vi "Obtain Request Events.vi"(8 "error in":errorcluster, 10 "Create New? (F)":bool) -> (0 "error out":errorcluster, 2 "Full User Interface Request Events":T1)   [LabVIEW 2019, in "Full User Interface.lvlib"]
doc: "This VI Obtains/Creates the Requests events that will be used for other modules to communicate with the module that owns this VI. These Requests events will be accessed only via Public API methods for this module.\n\n<b>NOTE</b>: The contents of this VI are automatically generated and modified by the <b>Tools > DQMH Consortium > DQMH</b> utilities. Consider using those utilities instead of making your own modifications to this VI.\n_____\nBased on DQMH Project Template 7.0.1.1316."
uses:
  Full User Interface.lvlib
  Request Events--cluster.ctl
  Stop Argument--cluster.ctl
  Show Panel Argument--cluster.ctl
  Hide Panel Argument--cluster.ctl
  Get Module Execution Status Argument--cluster.ctl
  Show Diagram Argument--cluster.ctl
  Launcher Test Unit Argument--cluster.ctl
  Exit Test Unit Argument--cluster.ctl
  Load Seq Argument--cluster.ctl
  Send UUT Result Argument--cluster.ctl
  Test Unit/UUT Result.ctl
  <vilib>/Test Bench Framework/Test Executive.lvlibp/TestEngine/TestEngine/TestEngine/Typedefs/Report General.ctl
  Send User Message Argument--cluster.ctl
  Change Model Argument--cluster.ctl
  <vilib>/Test Bench Framework/Test Executive.lvlibp/TestEngine/TestEngine/TestEngine/Test Engine.lvclass
  Test Unit/Test Unit.lvlib
panel:
  # "NOTE: The contents of this VI are automatically generated and modified by the Tools > DQMH Consortium > DQMH utilities. Consider using those utilities instead of making your own modifications to this VI."
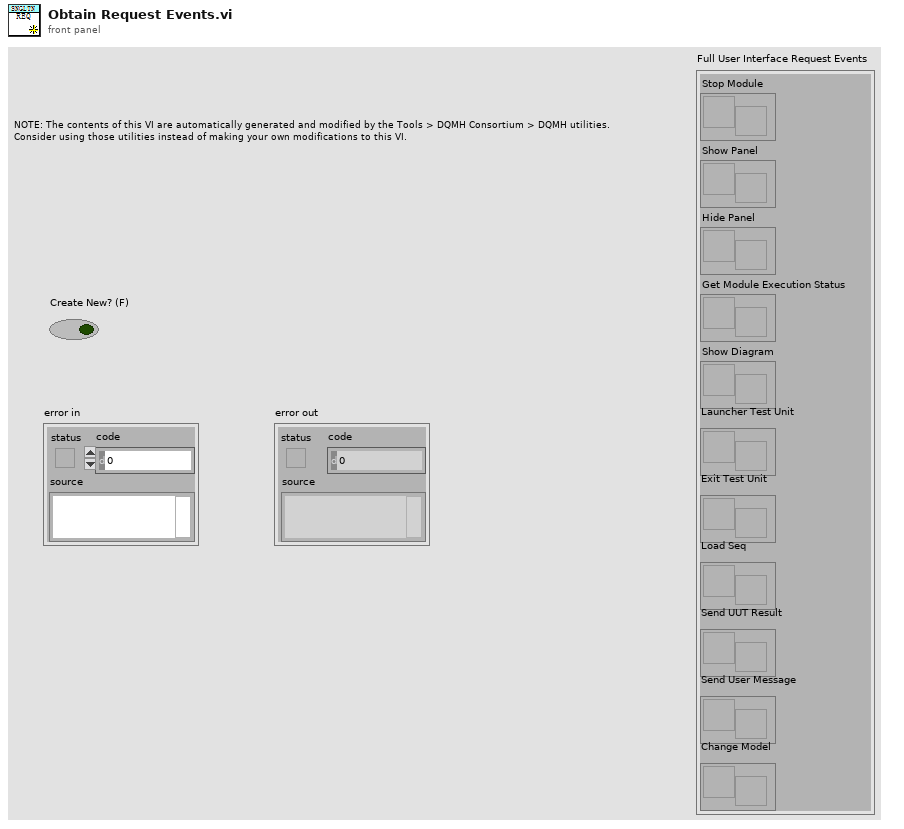
[diagram p1: front panel]
types:
  T1 = typedef "Full User Interface.lvlib/Request Events--cluster.ctl" = cluster{"Stop Module":refnum<user-event>, "Show Panel":refnum<user-event>, "Hide Panel":refnum<user-event>, "Get Module Execution Status":refnum<user-event>, "Show Diagram":refnum<user-event>, "Launcher Test Unit":refnum<user-event>, "Exit Test Unit":refnum<user-event>, "Load Seq":refnum<user-event>, "Send UUT Result":refnum<user-event>, "Send User Message":refnum<user-event>, "Change Model":refnum<user-event>}
  T2 = typedef "Full User Interface.lvlib/Change Model Argument--cluster.ctl" = cluster{"Model":string}
  T3 = typedef "Full User Interface.lvlib/Send User Message Argument--cluster.ctl" = cluster{"Station ID":i32, "Socket":i32, "UserMessage":string, "MessageData":variant}
  T4 = typedef "Full User Interface.lvlib/Send UUT Result Argument--cluster.ctl" = cluster{"UUT Result":T5, "Station":i32}
  T5 = typedef "Test Unit.lvlib/UUT Result.ctl" = cluster{"Station":i32, "Socket":i32, "DetailTestResult":string[][], "Report Path":path, "General":T6}
  T6 = typedef "Test Executive.lvlibp/Test Engine.lvlib/Test Engine.lvclass/Report General.ctl" = cluster{"Sequence Path":path, "Serial Number":string, "Test Date Time":timestamp, "UUT Status":string, "Faulty Item":string, "Seconds Executing":dbl}
  T7 = typedef "Full User Interface.lvlib/Load Seq Argument--cluster.ctl" = cluster{"Key":string}
  T8 = typedef "Full User Interface.lvlib/Exit Test Unit Argument--cluster.ctl" = cluster{"Checkbox":bool}
  T9 = typedef "Full User Interface.lvlib/Launcher Test Unit Argument--cluster.ctl" = cluster{"Checkbox":bool}
  T10 = typedef "Full User Interface.lvlib/Hide Panel Argument--cluster.ctl" = cluster{"Hide Panel?":bool}
  T11 = typedef "Full User Interface.lvlib/Show Panel Argument--cluster.ctl" = cluster{"Show Panel?":bool}
  T12 = typedef "Full User Interface.lvlib/Show Diagram Argument--cluster.ctl" = cluster{"Debug?":bool}
  T13 = typedef "Full User Interface.lvlib/Get Module Execution Status Argument--cluster.ctl" = cluster{"Running?":bool}
  T14 = typedef "Full User Interface.lvlib/Stop Argument--cluster.ctl" = cluster{"Origin":string, "Exit via Stop Module Req?":bool, "Wait for Module to stop?":bool}
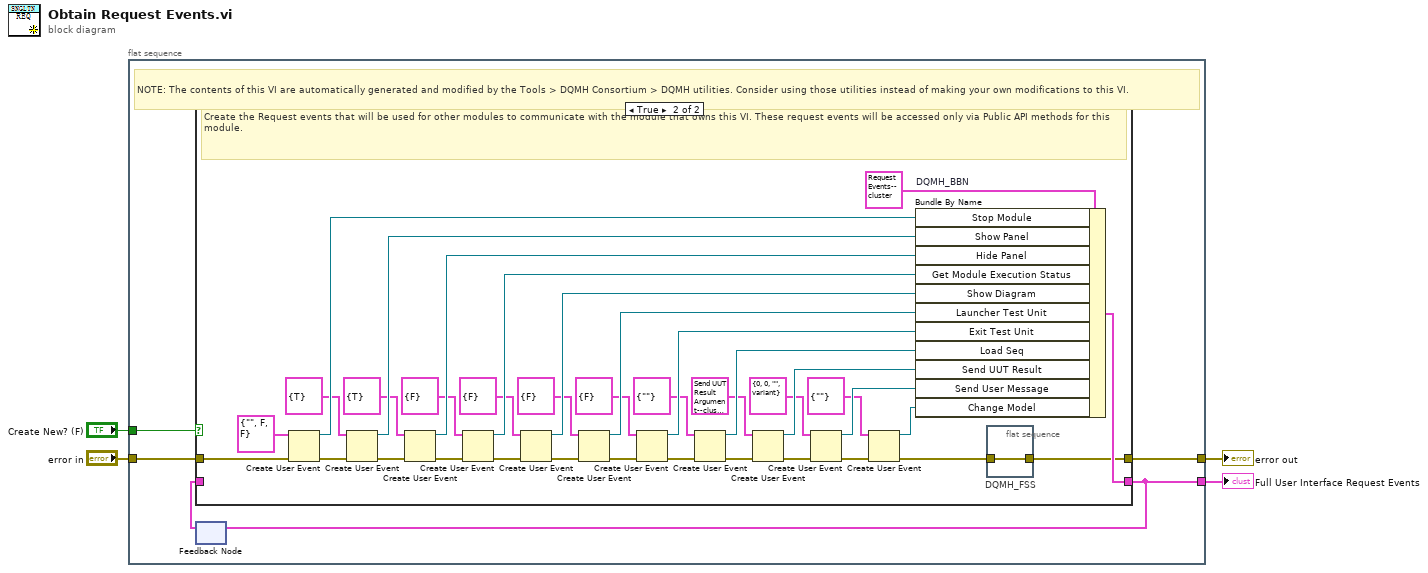
[diagram p0: block diagram]
diagram:
  n1 = flat-sequence {
    tunnel: [w9] -> w4
    tunnel: "error in" -> [w8]
    tunnel: [w6] -> w2
    tunnel: "Create New? (F)" -> [w5]
    frame #0 {
      # "NOTE: The contents of this VI are automatically generated and modified by the Tools > DQMH Consortium > DQMH utilities. Consider using those utilities instead of making your own modifications to this VI."
      n2 = feedback #1() -> (w7:T1)  [unwired: 1 in]
      n3 = case shown="True" w5 {
        tunnel: [w10 w38] -> w9
        tunnel: w8 -> [w10 w48]
        tunnel: [w11 w45] -> w6
        tunnel: w7 -> [w11 _]
        frame False {
          # "Obtain the Request events that were created in a previous call to this VI."
        }
        frame True {
          # "Create the Request events that will be used for other modules to communicate with the module that owns this VI. These request events will be accessed only via Public API methods for this module."
          n4 = Create User Event(user event datatype=T14 {"Origin"="", "Exit via Stop Module Req?"=FALSE, "Wait for Module to stop?"=FALSE} ("Stop Argument"), error in=w48) -> (user event=w46:refnum<user-event>, error out=w43:errorcluster)
          n5 = Create User Event(user event datatype=T11 {"Show Panel?"=TRUE} ("Show Panel Argument"), error in=w43) -> (user event=w42:refnum<user-event>, error out=w41:errorcluster)
          n6 = Create User Event(user event datatype=T10 {"Hide Panel?"=TRUE} ("Hide Panel Argument"), error in=w41) -> (user event=w40:refnum<user-event>, error out=w39:errorcluster)
          n7 = Create User Event(user event datatype=T13 {"Running?"=FALSE} ("Get Module Execution Status Argument"), error in=w39) -> (user event=w36:refnum<user-event>, error out=w37:errorcluster)
          n8 = Create User Event(user event datatype=T12 {"Debug?"=FALSE} ("Show Diagram Argument"), error in=w37) -> (user event=w33:refnum<user-event>, error out=w34:errorcluster)
          n9 = Create User Event(user event datatype=T9 {"Checkbox"=FALSE} ("Launcher Test Unit Argument"), error in=w34) -> (user event=w28:refnum<user-event>, error out=w29:errorcluster)
          n10 = Create User Event(user event datatype=T8 {"Checkbox"=FALSE} ("Exit Test Unit Argument"), error in=w29) -> (user event=w25:refnum<user-event>, error out=w26:errorcluster)
          n11 = Create User Event(user event datatype=T7 {"Key"=""} ("Load Seq Argument"), error in=w26) -> (user event=w22:refnum<user-event>, error out=w23:errorcluster)
          n12 = Create User Event(user event datatype=T4 {"UUT Result"={"Station"=0, "Socket"=0, "DetailTestResult"=[], "Report Path"=path "", "General"={"Sequence Path"=path "", "Serial Number"="", "Test Date Time"=timestamp(0 s since 1904-01-01), "UUT Status"="", "Faulty Item"="", "Seconds Executing"=0.0}}, "Station"=0} ("Send UUT Result Argument"), error in=w23) -> (user event=w19:refnum<user-event>, error out=w20:errorcluster)
          n13 = Create User Event(user event datatype=T3 {"Station ID"=0, "Socket"=0, "UserMessage"="", "MessageData"=variant(cluster{"Socket":i32, "UserMessage":string, "MessageData":variant} {"Socket"=0, "UserMessage"="", "MessageData"=variant})} ("Send User Message Argument"), error in=w20) -> (user event=w16:refnum<user-event>, error out=w17:errorcluster)
          n14 = Create User Event(user event datatype=T2 {"Model"=""} ("Change Model Argument"), error in=w17) -> (user event=w13:refnum<user-event>, error out=w14:errorcluster)
          n15 = Bundle By Name "DQMH_BBN"(cluster=T1 {"Stop Module"=refnum, "Show Panel"=refnum, "Hide Panel"=refnum, "Get Module Execution Status"=refnum, "Show Diagram"=refnum, "Launcher Test Unit"=refnum, "Exit Test Unit"=refnum, "Load Seq"=refnum, "Send UUT Result"=refnum, "Send User Message"=refnum, "Change Model"=refnum} ("output cluster"), "Stop Module"=w46, "Show Panel"=w42, "Hide Panel"=w40, "Get Module Execution Status"=w36, "Show Diagram"=w33, "Launcher Test Unit"=w28, "Exit Test Unit"=w25, "Load Seq"=w22, "Send UUT Result"=w19, "Send User Message"=w16, "Change Model"=w13) -> (w45:T1)
          n16 = flat-sequence "DQMH_FSS" {
            tunnel: w14 -> [w49]
            tunnel: [w49] -> w38
            frame #0 {
            }
          }
        }
      }
      n17 = feedback-in #1(w6) -> ()
    }
  }
  "Full User Interface Request Events" <- w2
  "error out" <- w4
